vi "Read_X_Y.vi"(8 "error in (no error)":errorcluster, 9 "Interface protocol":T1(ring), 10 "PIC Init?":bool, 11 "VISA resource name":refnum<visa-resource-name>) -> (0 "error out":errorcluster, 1 "Y":u32, 2 "X":u32, 3 "VISA resource name out":refnum<visa-resource-name>)   [LabVIEW 2017]
uses:
  <vilib>/Instr/_visa.llb/Select Event Type.ctl
  <vilib>/Instr/_visa.llb/VISA Configure Serial Port (Instr).vi
panel:
  out "FW Version":string
  out "read buffer":string
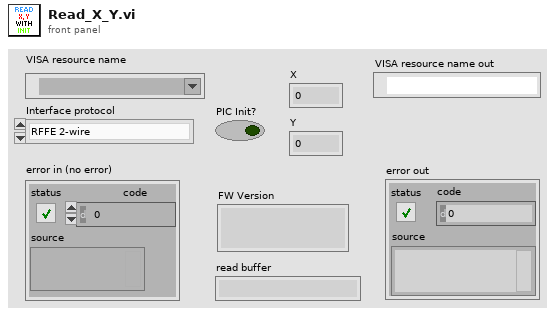
[diagram p1: front panel]
types:
  T1 = enum16{"RFFE 2-wire", "WiSPI 3-wire spi_sel", "WiSPI 4-wire spi_sel", "ifxSPI 3-wire spi_sel", "WiSPI 3-wire dev add spi_sel"}
  T2 = typedef "Select Event Type.ctl" = u32
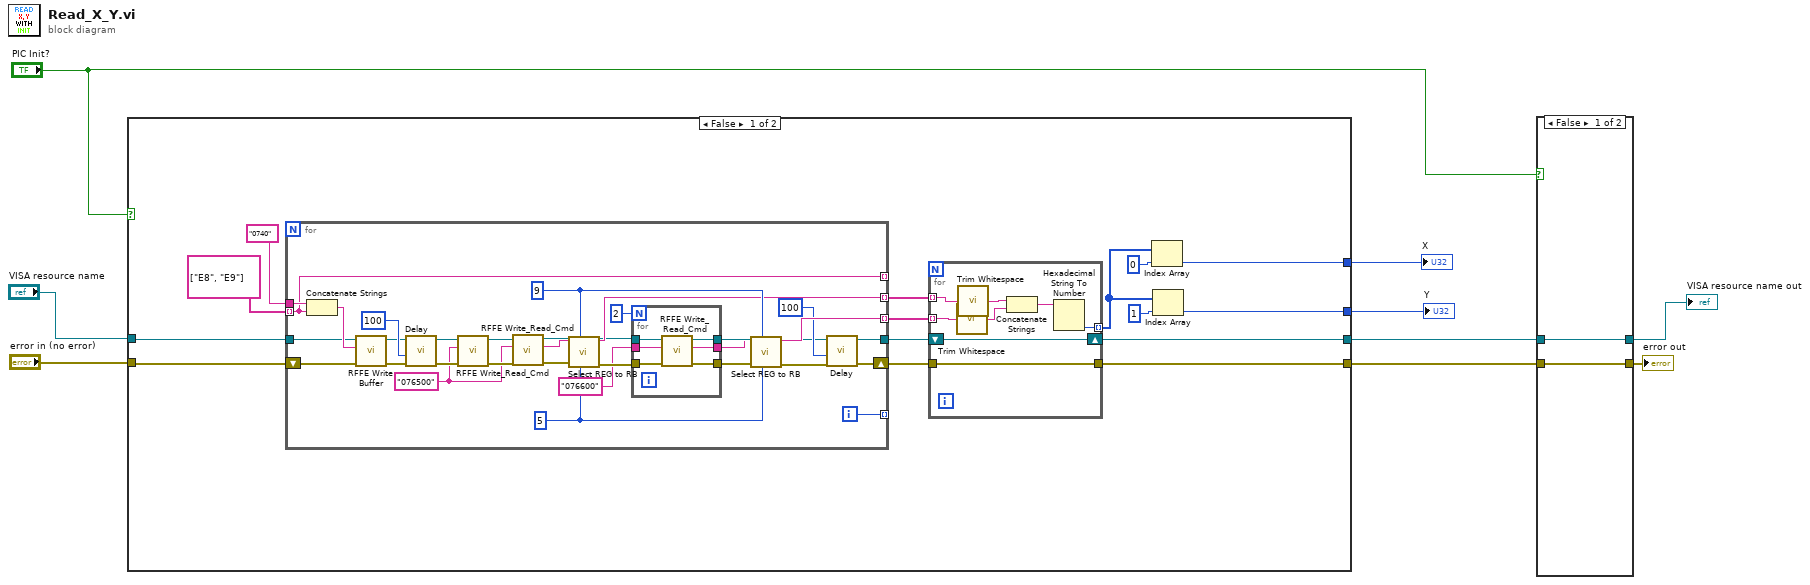
[diagram p0: block diagram]
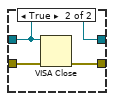
[diagram p2: hidden frame]
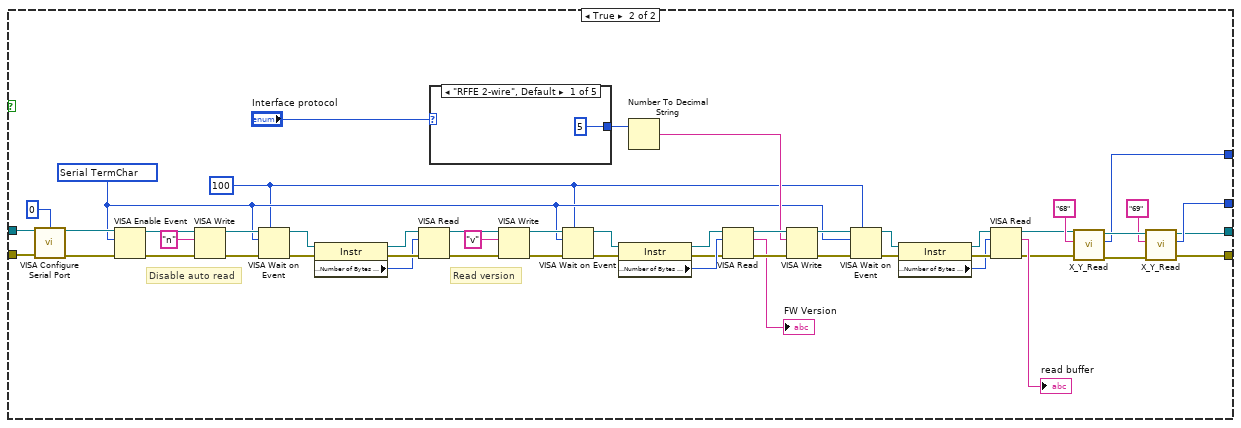
[diagram p3: hidden frame]
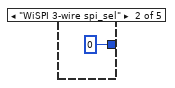
[diagram p4: hidden frame]
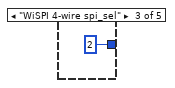
[diagram p5: hidden frame]
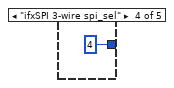
[diagram p6: hidden frame]
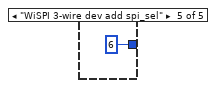
[diagram p7: hidden frame]
diagram:
  n1 = case shown="False" "PIC Init?" {
    tunnel: "error in (no error)" -> [w21 w83]
    tunnel: "VISA resource name" -> [w22 w82]
    tunnel: [w10 w69] -> w2
    tunnel: [w17 w68] -> w1
    tunnel: [w12 w73] -> w4
    tunnel: [w15 w72] -> w3
    frame False {
      n2 = for {
        shift-right: [w54] -> w18
        shift-left: w21 -> [w61]
        tunnel: string[] ["E8", "E9"] ("Add RB") -> [w52] mode=indexing
        tunnel: "0740" ("string") -> [w59]
        tunnel: [w56] -> w20 mode=indexing
        tunnel: [w55] -> w19 mode=indexing
        tunnel: [w52] -> _ mode=indexing
        tunnel: [w51] -> _ mode=indexing
        tunnel: [w42] -> w11
        tunnel: w22 -> [w41]
        i -> [w51]
        w37 = "076500" ("Cmd")
        w57 = 5 ("length")
        w58 = 9 ("offset")
        n3 = Concatenate Strings(w59, w52) -> (w60:string)
        n4 = call "RFFE Write Buffer.vi"("error in (no error)"=w61, "write buffer"=w60, "VISA resource name"=w41) -> ("error out"=w50:errorcluster, "VISA resource name out"=w47:refnum<visa-resource-name>)  [unwired: 7 in]
        n5 = call "Delay.vi"("error in (no error)"=w50, "Delay"=u32 100) -> ("error out"=w48:errorcluster)  [unwired: 9 in]
        n6 = call "RFFE Write_Read_Cmd.vi"("error in"=w48, "Cmd"=w37, "VISA In"=w47) -> ("error out"=w39:errorcluster, "VISA Out"=w38:refnum<visa-resource-name>)  [unwired: 6 in, 1 out]
        n7 = call "RFFE Write_Read_Cmd.vi"("error in"=w39, "Cmd"=w37, "VISA In"=w38) -> ("error out"=w36:errorcluster, "read buffer"=w35:string, "VISA Out"=w34:refnum<visa-resource-name>)  [unwired: 6 in]
        n8 = call "Select REG to RB.vi"("length"=w57, "offset"=w58, "Error In"=w36, "Manual Write"=w35) -> ("Error Out"=w45:errorcluster, "Readback"=w56:string)  [unwired: 6 in]
        n9 = for {
          N: 2 -> [_]
          tunnel: "076600" ("Cmd") -> [w67]
          tunnel: w45 -> [w66]
          tunnel: w34 -> [w65]
          tunnel: [w64] -> w42
          tunnel: [w63] -> w46
          tunnel: [w62] -> w40
          n10 = call "RFFE Write_Read_Cmd.vi"("error in"=w66, "Cmd"=w67, "VISA In"=w65) -> ("error out"=w63:errorcluster, "read buffer"=w62:string, "VISA Out"=w64:refnum<visa-resource-name>)  [unwired: 6 in]
        }
        n11 = call "Select REG to RB.vi"("length"=w57, "offset"=w58, "Error In"=w46, "Manual Write"=w40) -> ("Error Out"=w33:errorcluster, "Readback"=w55:string)  [unwired: 6 in]
        n12 = call "Delay.vi"("error in (no error)"=w33, "Delay"=u32 100) -> ("error out"=w54:errorcluster)  [unwired: 9 in]
      }
      n13 = for {
        tunnel: w20 -> [w32] mode=indexing
        tunnel: w19 -> [w31] mode=indexing
        tunnel: [w30] -> w13 mode=indexing
        tunnel: w18 -> [w29]
        tunnel: [w29] -> w17
        shift-right: [w28] -> w10
        shift-left: w11 -> [w28]
        n14 = call <vilib>:"Trim Whitespace.vi"("string"=w31) -> ("trimmed string"=w25:string)  [unwired: 1 in]
        n15 = call <vilib>:"Trim Whitespace.vi"("string"=w32) -> ("trimmed string"=w26:string)  [unwired: 1 in]
        n16 = Concatenate Strings(w26, w25) -> (w27:string)
        n17 = Hexadecimal String To Number(string=w27) -> (number=w30:u32)  [unwired: 2 in, 1 out]
      }
      n18 = Index Array(array=w13, index=0) -> (element=w15:u32)
      n19 = Index Array(array=w13, index=1) -> (element=w12:u32)
    }
    frame True {
      w79 = u32 100 ("timeout (0)")
      w80 = T2 1073684516 items=["Service Request"=1073684491, "Trigger"=3221168138, "Clear"=1073684493, "VXI Signal"=1073684512, "VXI/VME Interrupt"=3221168161, "VXI/VME Sysfail"=1073684509, "VXI/VME Sysreset"=1073684510, "GPIB CIC"=1073684498, "GPIB Talk"=1073684499, "GPIB Listen"=1073684500, "PXI Interrupt"=1073684514, "Serial Break"=1073684515, "Serial TermChar"=1073684516, "Serial CTS"=1073684521, "Serial DSR"=1073684522, "Serial DCD"=1073684524, "Serial RI"=1073684526, "Serial Character"=1073684533, "USB Interrupt"=1073684535, "All Enabled"=1073709055] ("Event Type")
      # "Read version"
      # "Disable auto read"
      n20 = call-poly "VISA Configure Serial Port"("VISA resource name"=w82, "termination char\n(0xA = '\\n' = LF)"=u8 0 ("termination char\n(0xA = '\\n' = LF)"), "error in (no error)"=w83) -> ("VISA resource name out"=w116:refnum<visa-resource-name>, "error out"=w117:errorcluster)  [unwired: 11 in]
      n21 = VISA Enable Event(8:w117, 10:w80, 11:w116) -> (0:w115:errorcluster, 3:w114:refnum<visa-resource-name>)  [unwired: 1 in]
      n22 = VISA Write(VISA resource name=w114, write buffer="n", error in (no error)=w115) -> (VISA resource name out=w111:refnum<visa-resource-name>, error out=w112:errorcluster)  [unwired: 1 out]
      n23 = VISA Wait on Event(7:w79, 8:w112, 10:w80, 11:w111) -> (0:w109:errorcluster, 3:w110:refnum<visa-resource-name>)  [unwired: 1 in, 2 out]
      n24 = property class="Instr"(reference=w110, error in=w109) -> (reference out=w106:refnum<visa-resource-name>, error out=w108:errorcluster, "Serial Settings:Number of Bytes at Serial Port"=w107:u32)
      n25 = VISA Read(VISA resource name=w106, byte count=w107, error in (no error)=w108) -> (VISA resource name out=w90:refnum<visa-resource-name>, error out=w89:errorcluster)  [unwired: 2 out]
      n26 = case shown="\"RFFE 2-wire\", Default" "Interface protocol" {
        tunnel: [5 0 2 4 6] -> w86
        frame "RFFE 2-wire", Default {
        }
        frame "WiSPI 3-wire spi_sel" {
        }
        frame "WiSPI 4-wire spi_sel" {
        }
        frame "ifxSPI 3-wire spi_sel" {
        }
        frame "WiSPI 3-wire dev add spi_sel" {
        }
      }
      n27 = VISA Write(VISA resource name=w90, write buffer="v", error in (no error)=w89) -> (VISA resource name out=w93:refnum<visa-resource-name>, error out=w92:errorcluster)  [unwired: 1 out]
      n28 = VISA Wait on Event(7:w79, 8:w92, 10:w80, 11:w93) -> (0:w95:errorcluster, 3:w94:refnum<visa-resource-name>)  [unwired: 1 in, 2 out]
      n29 = property class="Instr"(reference=w94, error in=w95) -> (reference out=w98:refnum<visa-resource-name>, error out=w96:errorcluster, "Serial Settings:Number of Bytes at Serial Port"=w97:u32)
      n30 = Number To Decimal String(number=w86) -> (decimal integer string=w85:string)  [unwired: 1 in]
      n31 = VISA Read(VISA resource name=w98, byte count=w97, error in (no error)=w96) -> (VISA resource name out=w87:refnum<visa-resource-name>, read buffer=→"FW Version":string, error out=w88:errorcluster)  [unwired: 1 out]
      n32 = VISA Write(VISA resource name=w87, write buffer=w85, error in (no error)=w88) -> (VISA resource name out=w104:refnum<visa-resource-name>, error out=w105:errorcluster)  [unwired: 1 out]
      n33 = VISA Wait on Event(7:w79, 8:w105, 10:w80, 11:w104) -> (0:w102:errorcluster, 3:w103:refnum<visa-resource-name>)  [unwired: 1 in, 2 out]
      n34 = property class="Instr"(reference=w103, error in=w102) -> (reference out=w99:refnum<visa-resource-name>, error out=w101:errorcluster, "Serial Settings:Number of Bytes at Serial Port"=w100:u32)
      n35 = VISA Read(VISA resource name=w99, byte count=w100, error in (no error)=w101) -> (VISA resource name out=w70:refnum<visa-resource-name>, read buffer=→"read buffer":string, error out=w71:errorcluster)  [unwired: 1 out]
      n36 = call "X_Y_Read.vi"("error in (no error)"=w71, "Address to Read"="68", "VISA resource name In"=w70) -> ("error out"=w76:errorcluster, "Number Out"=w72:u32, "VISA resource name out"=w77:refnum<visa-resource-name>)  [unwired: 6 in]
      n37 = call "X_Y_Read.vi"("error in (no error)"=w76, "Address to Read"="69", "VISA resource name In"=w77) -> ("error out"=w68:errorcluster, "Number Out"=w73:u32, "VISA resource name out"=w69:refnum<visa-resource-name>)  [unwired: 6 in]
    }
  }
  "Y" <- w4
  "X" <- w3
  n38 = case shown="False" "PIC Init?" {
    tunnel: [w125 w128] -> w7
    tunnel: w2 -> [w124 w126]
    tunnel: w1 -> [w125 w127]
    tunnel: [w124 w126] -> w5
    frame False {
    }
    frame True {
      n39 = VISA Close(VISA resource name=w126, error in (no error)=w127) -> (error out=w128:errorcluster)
    }
  }
  "error out" <- w7
  "VISA resource name out" <- w5
